vi "참조 생성하기 2.vi"() -> ()   [LabVIEW 2020]
panel:
  in  "숫자형":dbl
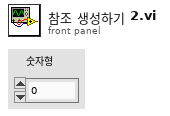
[diagram p1: front panel]
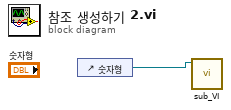
[diagram p0: block diagram]
diagram:
  n1 = control-ref of="숫자형"() -> (w1:refnum<vi>)
  n2 = call "sub_VI.vi"("Ctl 참조 번호"=w1) -> ()  [unwired: 11 in]
